vi "Left LIDAR Loop (SubVI).vi"(11 "Refnum in":refnum<k20>) -> ()   [LabVIEW 2015]
uses:
  Left Variables.vi
  <vilib>/Utility/error.llb/Error Cluster From Error Code.vi
  <vilib>/rvi/errors/niLvFpgaAdjustHostInterfaceError.vi
  <vilib>/FPGAPlugInAG/Dynamic/niLvFpga_Close_Dynamic.vi
  <vilib>/rvi/interface/nirviReadWriteControl/nirviReadWriteControl.xnode
  <vilib>/rvi/interface/nirviCloseFPGA/nirviCloseFPGA.xnode
  NiFpgaLv.dll
  <vilib>/rvi/interface/Simulation/niFpgaSimulationCallBeginRW.vi
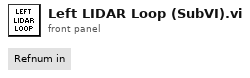
[diagram p1: front panel]
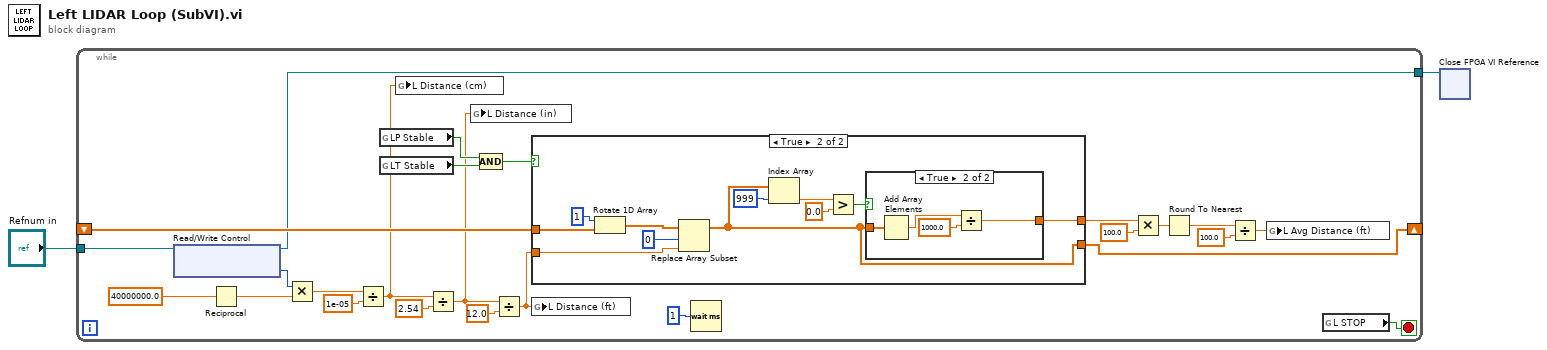
[diagram p0: block diagram]
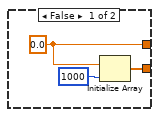
[diagram p2: hidden frame]
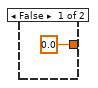
[diagram p3: hidden frame]
diagram:
  n1 = while {
    tunnel: "Refnum in" -> [w8]
    tunnel: [w7] -> w2
    shift-right: [w24] -> _
    shift-left: _ -> [w23]
    stop <- w3 stop-if-true
    n2 = xnode "Read/Write Control"("FPGA VI Reference In"=w8) -> ("FPGA VI Reference Out"=w7:refnum<k20>, "Pulse width ticks"=w11:u32)  [unwired: 1 in, 1 out]
    n3 = Reciprocal(x=40000000.0) -> (1/x=w10:dbl)
    n4 = Multiply(x=w11, y=w10) -> (x*y=w12:dbl)
    n5 = Divide(x=w12, y=1e-05) -> (x/y=w6:dbl)
    n6 = global read "Left Variables.vi" "LP Stable"() -> (w26:bool)
    n7 = global read "Left Variables.vi" "LT Stable"() -> (w27:bool)
    n8 = global write "Left Variables.vi" "L Distance (cm)"(w6) -> ()
    n9 = Divide(x=w6, y=2.54) -> (x/y=w5:dbl)
    n10 = global write "Left Variables.vi" "L Distance (in)"(w5) -> ()
    n11 = Compound Arithmetic op=AND(w26, w27) -> (w25:bool)
    n12 = Divide(x=w5, y=12.0) -> (x/y=w4:dbl)
    n13 = case shown="True" w25 {
      tunnel: w23 -> [_ w34]
      tunnel: [w28 w32] -> w24
      tunnel: [w29 w33] -> w22
      tunnel: w4 -> [_ w31]
      frame False {
        w29 = 0.0 ("element")
        n14 = Initialize Array(w29, 1000 ("dimension size")) -> (w28:dbl[])
      }
      frame True {
        n15 = Rotate 1D Array(1:w34, 2:1 ("n")) -> (0:w40:dbl[])
        n16 = Replace Array Subset(array=w40, new element=w31, index=0) -> (w32:dbl[])
        n17 = Index Array(array=w32, index=999) -> (element=w37:dbl)
        n18 = Greater?(x=w37, y=0.0) -> (0:w35:bool)
        n19 = case shown="True" w35 {
          tunnel: w32 -> [_ w46]
          tunnel: [0.0 w43] -> w33
          frame False {
          }
          frame True {
            n20 = Add Array Elements(numeric array=w46) -> (sum=w45:dbl)
            n21 = Divide(x=w45, y=1000.0) -> (x/y=w43:dbl)
          }
        }
      }
    }
    n22 = global write "Left Variables.vi" "L Distance (ft)"(w4) -> ()
    n23 = Wait (ms)(milliseconds to wait=u32 1) -> ()  [unwired: 1 out]
    n24 = Multiply(x=w22, y=100.0) -> (x*y=w20:dbl)
    n25 = Round To Nearest(number=w20) -> (nearest integer value=w19:dbl)
    n26 = Divide(x=w19, y=100.0) -> (x/y=w17:dbl)
    n27 = global write "Left Variables.vi" "L Avg Distance (ft)"(w17) -> ()
    n28 = global read "Left Variables.vi" "L STOP"() -> (w3:bool)
  }
  n29 = xnode "Close FPGA VI Reference"("FPGA VI Reference In"=w2) -> ()  [unwired: 1 in, 1 out]
